vi "postScanHoldtime.vi"(6 "Settling Time":dbl[unit], 9 "Sample Count":u32, 10 "ILC Rate":dbl[unit], 11 "Delta":dbl) -> (2 "PostScan Hold time":dbl[unit], 3 "Boolean":bool)   [LabVIEW 2015]
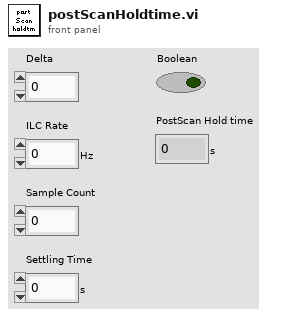
[diagram p1: front panel]
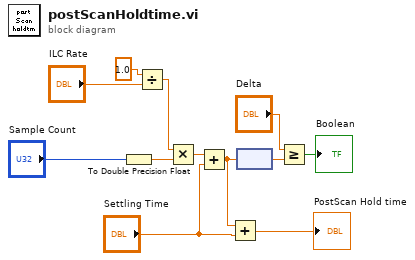
[diagram p0: block diagram]
diagram:
  n1 = To Double Precision Float(number="Sample Count") -> (double precision float=w7:dbl)
  n2 = Divide(x=1.0, y="ILC Rate") -> (x/y=w6:dbl[unit])
  n3 = Multiply(x=w6, y=w7) -> (x*y=w9:dbl[unit])
  n4 = Add(x=w9, y="Settling Time") -> (x+y=w3:dbl[unit])
  n5 = Add(x=w3, y="Settling Time") -> (x+y=→"PostScan Hold time":dbl[unit])
  n6 = node(w3) -> (w11:dbl)
  n7 = Greater Or Equal?(x="Delta", y=w11) -> (x >= y?=→"Boolean":bool)
